vi "test_Export Instrument Addon Config.vi"(8 "error in (no error)":errorcluster, 11 "TestCase in":refnum<class "Instrument Addon Scripting API Custom Device Unit Tests.lvclass">) -> (0 "error out":errorcluster, 3 "TestCase out":refnum<class "Instrument Addon Scripting API Custom Device Unit Tests.lvclass">)   [LabVIEW 2018, in "Instrument Addon Scripting API Custom Device Unit Tests.lvclass"]
uses:
  Instrument Addon Scripting API Custom Device Unit Tests.lvclass
  NationalInstruments.VeriStand.SystemDefinitionAPI
  Instrument Addon Scripting API Custom Device Unit Tests.lvclass/Instrument Addon Scripting API Custom Device Unit Tests.ctl
  Addon/Addon Shared/SubVIs/Constants.vi
  <vilib>/NI Veristand/Custom Device Tools/Custom Device Utility Library/NI VeriStand - Search for Item by GUID.vi
  <vilib>/addons/_JKI Toolkits/VI Tester/TestCase.llb/TestCase.lvclass
  Instrument Addon Scripting API Test Assets/Instrument Addon Scripting API Test Assets.lvclass
  APIs/Scripting API/Instrument Addon Scripting API.lvlib
  <vilib>/NI Veristand/Custom Device Tools/Custom Device Utility Library/Custom Device Utility Library.lvlib
  Addon/Addon Shared/Instrument Addon Shared.lvlib
  C:/Program Files (x86)/National Instruments/LabVIEW 2018/vi.lib/addons/_JKI Toolkits/VI Tester/TestCase.llb/TestCase.lvclass
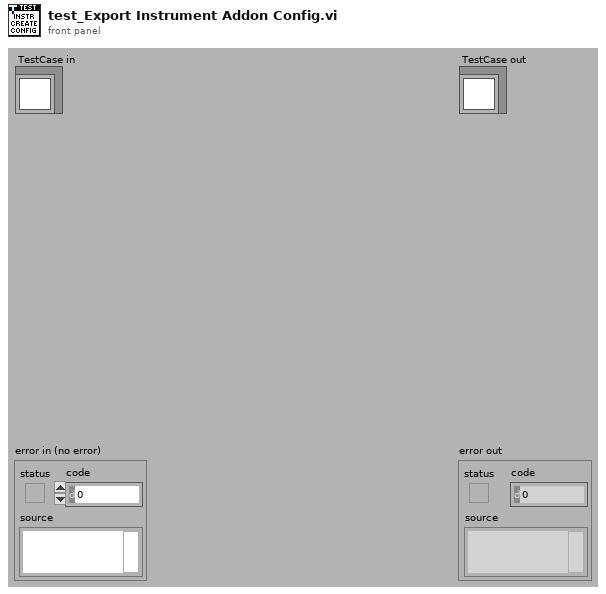
[diagram p1: front panel]
types:
  T1 = typedef "Custom Device API.lvlib/Custom Device Item Ref.ctl" = u64
  T2 = cluster{"Message Group Ref":T1, "Message Channels Refs":T1[]}[]
  T3 = cluster{"Message Group Ref":T1, "Message Channels Refs":T1[]}
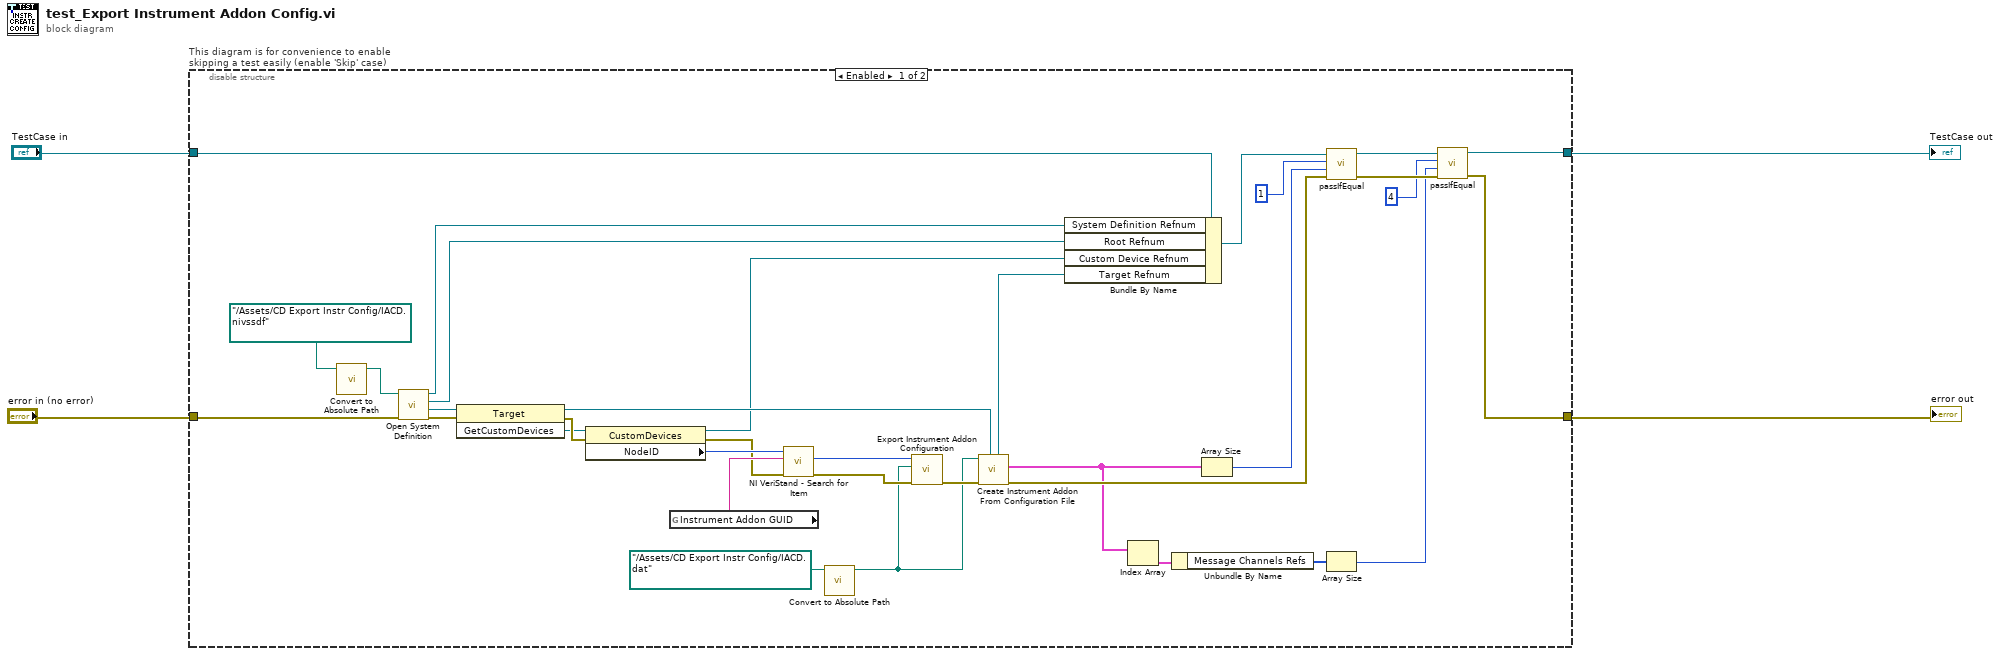
[diagram p0: block diagram]
diagram:
  n1 = disable-structure "This diagram is for convenience to enable skipping a test easily (enable 'Skip' case)" shown="Enabled" {
    disable-tunnel: "TestCase in" -> [w10 w42]
    disable-tunnel: [w17 w40] -> w1
    disable-tunnel: [w11 w41] -> w3
    disable-tunnel: "error in (no error)" -> [w38 w39]
    frame Enabled {
      n2 = call "Convert to Absolute Path.vi"("System Definition File"=path "../Assets/CD Export Instr Config/IACD.nivssdf" ("SDF file")) -> ("Absolute Path"=w36:path)  [unwired: 10 in]
      n3 = call "Open System Definition.vi"("error in (no error)"=w38, "System Definition File"=w36) -> ("error out"=w32:errorcluster, "Target Refnum"=w31:refnum<k24>, "Root Refnum"=w7:refnum<k24>, "System Definition Refnum"=w8:refnum<k24>)  [unwired: 6 in]
      n4 = invoke class="Target" method="GetCustomDevices"(reference=w31, error in=w32) -> (reference out=w23:refnum<k24>, error out=w34:errorcluster, "GetCustomDevices"=w33:refnum<k24>)  [unwired: 1 in]
      n5 = property class="CustomDevices"(reference=w33, error in=w34) -> (reference out=w6:refnum<k24>, error out=w28:errorcluster, "NodeID"=w30:u64)
      n6 = global read "Constants.vi" "Instrument Addon GUID"() -> (w29:string)
      n7 = call-poly <vilib>:"NI VeriStand - Search for Item.vi"("error in"=w28, "Item GUID"=w29, "Section Ref in"=w30) -> ("error out"=w27:errorcluster, "Item Ref"=w26:T1)  [unwired: 5 in, 2 out]
      n8 = call "Convert to Absolute Path.vi"("System Definition File"=path "../Assets/CD Export Instr Config/IACD.dat" ("SDF file")) -> ("Absolute Path"=w24:path)  [unwired: 10 in]
      n9 = call "Export Instrument Addon Configuration.vi"("error in (no error)"=w27, "Exported File Path"=w24, "Instrument Addon Refnum In"=w26) -> ("error out"=w25:errorcluster)  [unwired: 7 in, 1 out]
      n10 = call "Create Instrument Addon From Configuration File.vi"("Target in"=w23, "error in (no error)"=w25, "CD Config Path (.dat)"=w24) -> ("error out"=w22:errorcluster, "Message Channels refnums"=w15:T2, "Target out"=w5:refnum<k24>)  [unwired: 5 in, 1 out]
      n11 = Bundle By Name(cluster=w10, "System Definition Refnum"=w8, "Root Refnum"=w7, "Custom Device Refnum"=w6, "Target Refnum"=w5) -> (w9:refnum<class "Instrument Addon Scripting API Custom Device Unit Tests.lvclass">)
      n12 = Index Array(array=w15) -> (element=w14:T3)  [unwired: 1 in]
      n13 = Unbundle By Name(w14) -> ("Message Channels Refs"=w13:T1[])
      n14 = Array Size(array=w15) -> (size(s)=w16:i32)
      n15 = call-dynamic "passIfEqual.vi"("error in (no error)"=w22, "y"=w16, "x"=1 ("size(s)"), "TestCase in"=w9) -> ("error out"=w20:errorcluster, "TestCase out"=w21:refnum<class "Instrument Addon Scripting API Custom Device Unit Tests.lvclass">)  [unwired: 6 in]
      n16 = Array Size(array=w13) -> (size(s)=w12:i32)
      n17 = call-dynamic "passIfEqual.vi"("error in (no error)"=w20, "y"=w12, "x"=4 ("size(s)"), "TestCase in"=w21) -> ("error out"=w11:errorcluster, "TestCase out"=w17:refnum<class "Instrument Addon Scripting API Custom Device Unit Tests.lvclass">)  [unwired: 6 in]
    }
    frame Disabled {
      # "skip test result while test is under development"
      n18 = call <vilib>:"skip.vi"("error in (no error)"=w39, "TestCase in"=w42) -> ("error out"=w41:errorcluster, "TestCase out"=w40:refnum<class "Instrument Addon Scripting API Custom Device Unit Tests.lvclass">)  [unwired: 8 in]
    }
  }
  "error out" <- w3
  "TestCase out" <- w1
